vi "Set FFT Size.vi"(8 "error in (no error)":errorcluster, 10 "FFT Size":T1={"FFT Size"=1048576}, 11 "Signal Analysis in":refnum<class "Signal Analysis.lvclass">) -> (0 "error out":errorcluster, 3 "Signal Analysis out":refnum<class "Signal Analysis.lvclass">)   [LabVIEW 2025, in "Signal Analysis.lvlib" / "Signal Analysis.lvclass"]
uses:
  Signal Analysis.lvclass
  Signal Analysis.lvclass/Signal Analysis.ctl
  Helper Loop Type.ctl
  Helper Loop Message.ctl
  FFT Size.ctl
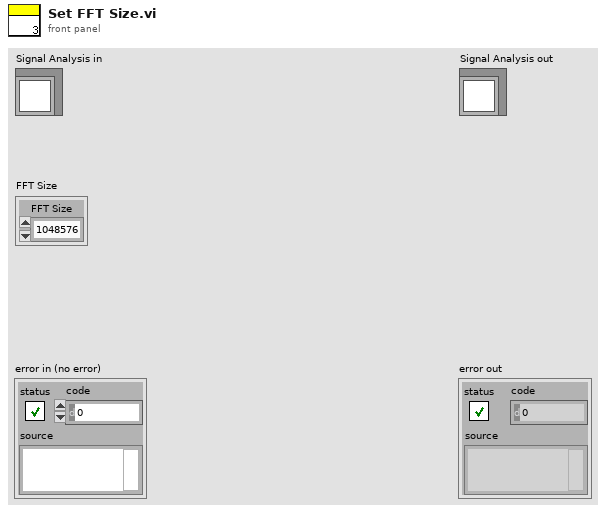
[diagram p1: front panel]
types:
  T1 = typedef "Signal Analysis.lvlib/Signal Analysis.lvclass/FFT Size.ctl" = cluster{"FFT Size":i32}
  T2 = typedef "Signal Analysis.lvlib/Signal Analysis.lvclass/Helper Loop Message.ctl" = cluster{"Type":T3, "Payload":variant}
  T3 = typedef "Signal Analysis.lvlib/Signal Analysis.lvclass/Helper Loop Type.ctl" = enum16{"Process Data", "Set Render Prio", "Close", "Set FFT Size"}
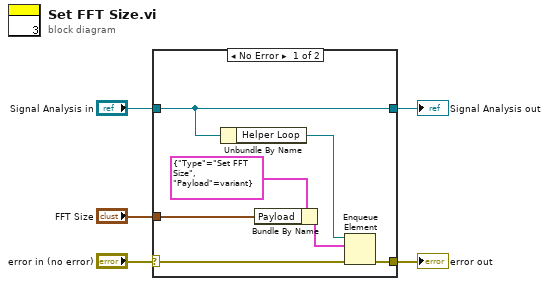
[diagram p0: block diagram]
diagram:
  n1 = case shown="No Error" "error in (no error)" {
    selector: "error in (no error)" -> [w8 w14]
    tunnel: [w7 w14] -> w4
    tunnel: [w9 w13] -> w2
    tunnel: "Signal Analysis in" -> [w9 w13]
    tunnel: "FFT Size" -> [w6 _]
    frame No Error {
      n2 = Unbundle By Name(w9) -> ("Helper Loop"=w11:refnum<queue>)
      n3 = Bundle By Name(cluster=T2 {"Type"=enum."Set FFT Size", "Payload"=variant} ("element"), "Payload"=w6) -> (w12:T2)
      n4 = Enqueue Element(queue=w11, element=w12, error in (no error)=w8) -> (error out=w7:errorcluster)  [unwired: 1 in, 2 out]
    }
    frame Error {
    }
  }
  "error out" <- w4
  "Signal Analysis out" <- w2
